vi "prova1.vi"() -> ()   [LabVIEW 2013]
panel:
  in  "Plot.Plot Name":string
  in  "Y Scale.Name Label.Text":string
  in  "Plot.Y Scale Index 2":u32
  in  "Y Scale.Range:Minimum":dbl
  in  "Y Scale.Range:Maximum":dbl
  out "Strip Chart":cluster{dbl, dbl}(graph)={0.6048539044559809, 0.9356575577636529}
  in  "Tab Control":enum32{"Analisi Dati", "Page 2", "Page 3"}(tab)
  out "Waveform Chart":dbl(graph)
  out "Waveform Graph":dbl[](graph)
  out "Connesso?":bool
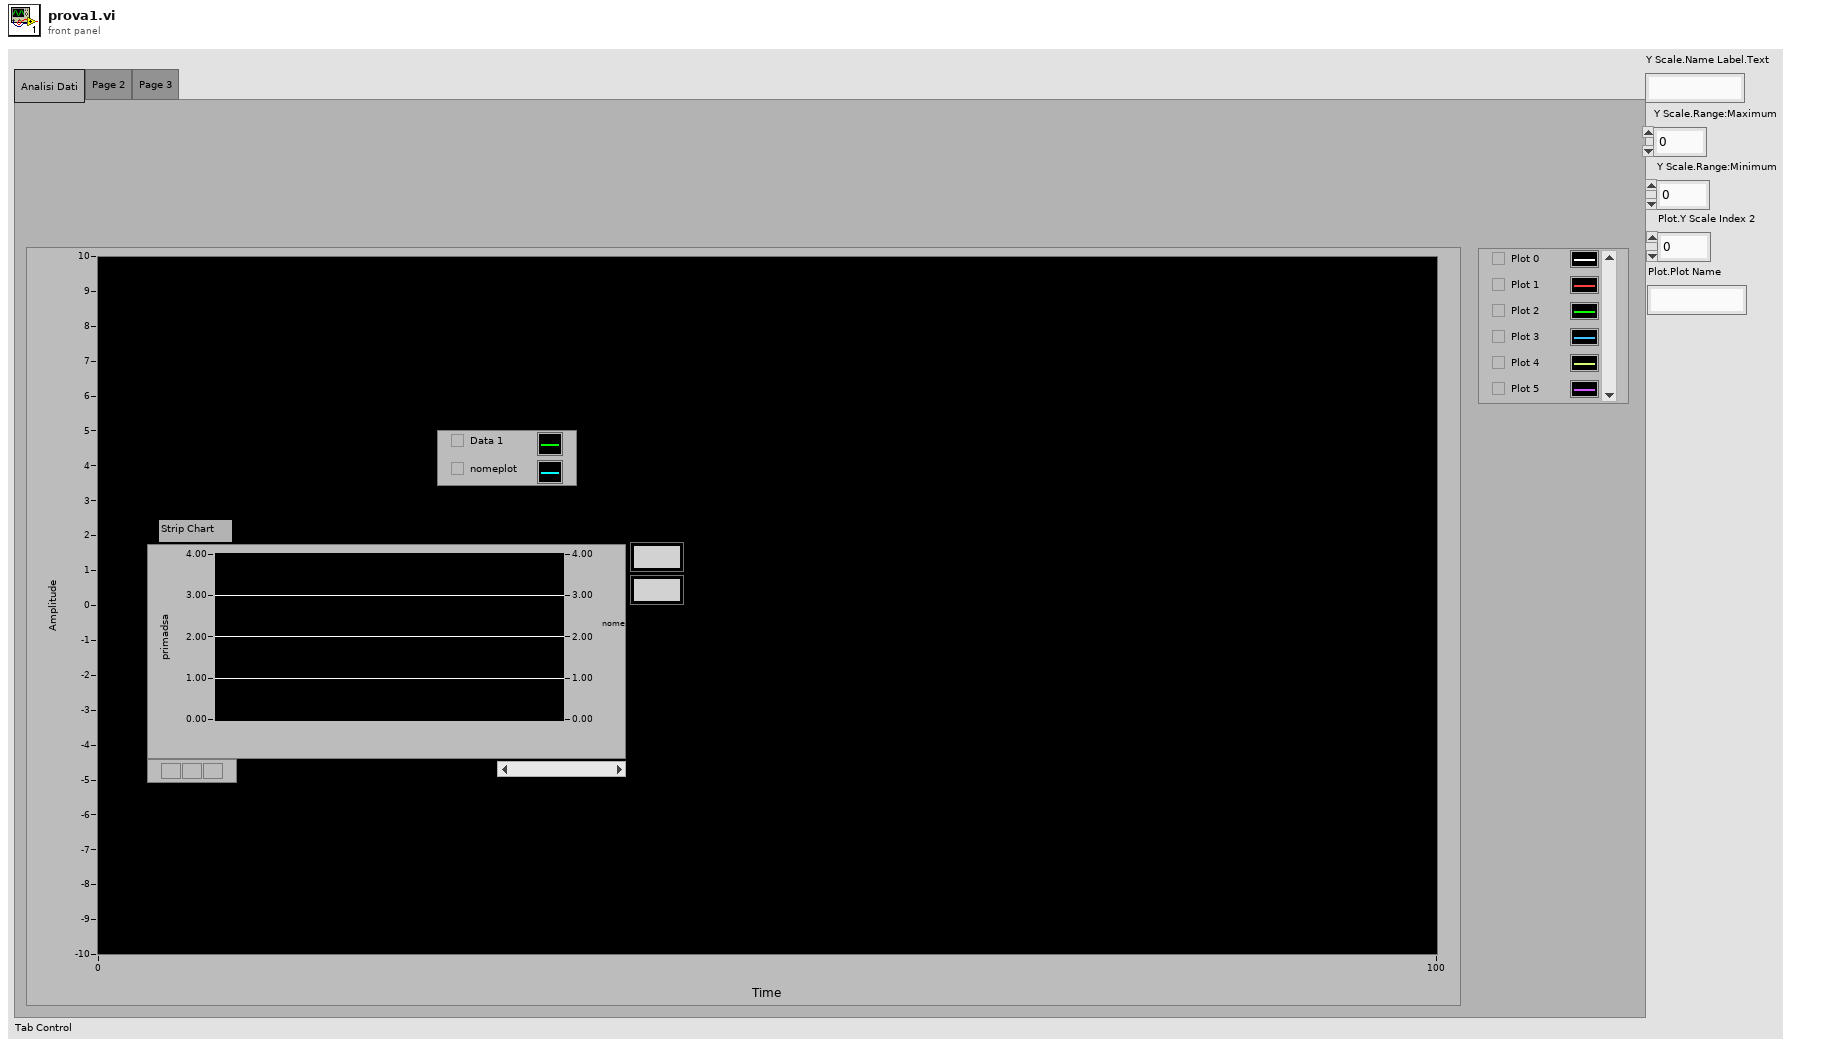
[diagram p1: front panel]
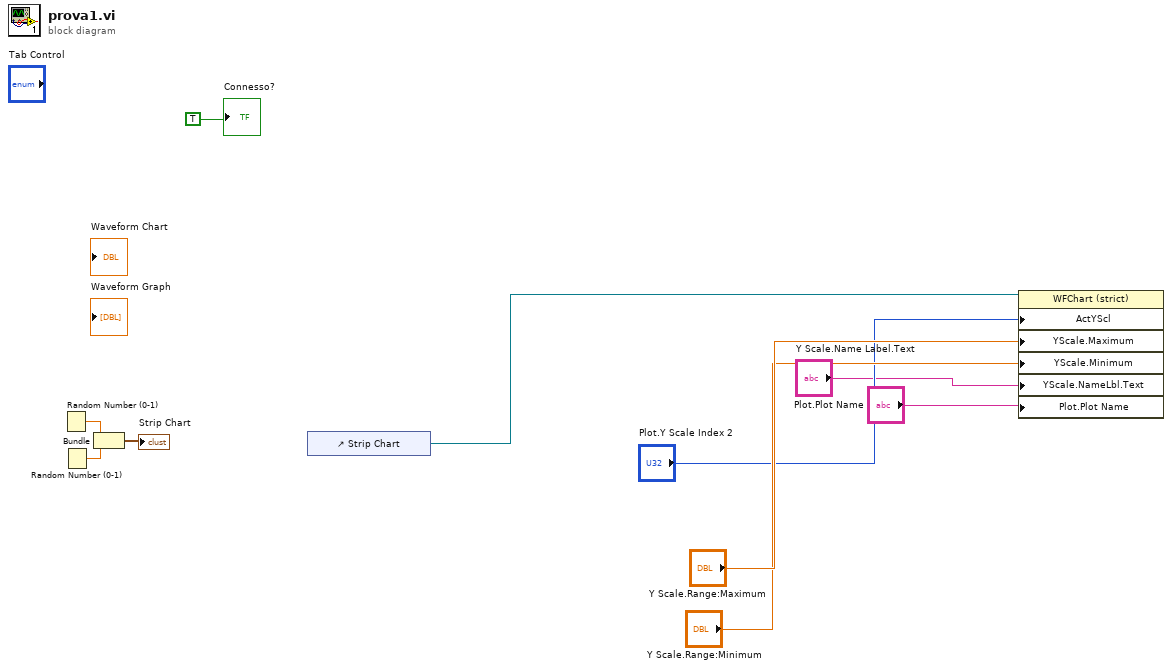
[diagram p0: block diagram]
diagram:
  n1 = Random Number (0-1)() -> (number: 0 to 1=w9:dbl)
  n2 = Random Number (0-1)() -> (number: 0 to 1=w10:dbl)
  n3 = Bundle(w9, w10) -> (→"Strip Chart":cluster{dbl, dbl})  [unwired: 1 in]
  n4 = control-ref of="Strip Chart"() -> (w7:refnum<vi>)
  n5 = property class="WFChart (strict)"(reference=w7, "ActYScl"="Plot.Y Scale Index 2", "YScale.Maximum"="Y Scale.Range:Maximum", "YScale.Minimum"="Y Scale.Range:Minimum", "YScale.NameLbl.Text"="Y Scale.Name Label.Text", "Plot.Plot Name"="Plot.Plot Name") -> ()  [unwired: 1 in, 2 out]
  "Connesso?" <- TRUE
